vi "Create Humi Tag.vi"(8 "error in (no error)":errorcluster, 11 "CVT Tags to Create":T1) -> (0 "error out":errorcluster, 3 "CVT CFG Out":T1)   [LabVIEW 2016, in "CVT.lvlib"]
uses:
  <vilib>/NI/Current Value Table/Type Defs/File Format.ctl
  <vilib>/NI/Current Value Table/Type Defs/Single Tag.ctl
  <vilib>/NI/Current Value Table/Type Defs/Data Types.ctl
  <vilib>/NI/Current Value Table/Type Defs/Tag Grouping set.ctl
  CVT.lvlib
  <vilib>/NI/Current Value Table/Current Value Table.lvlib
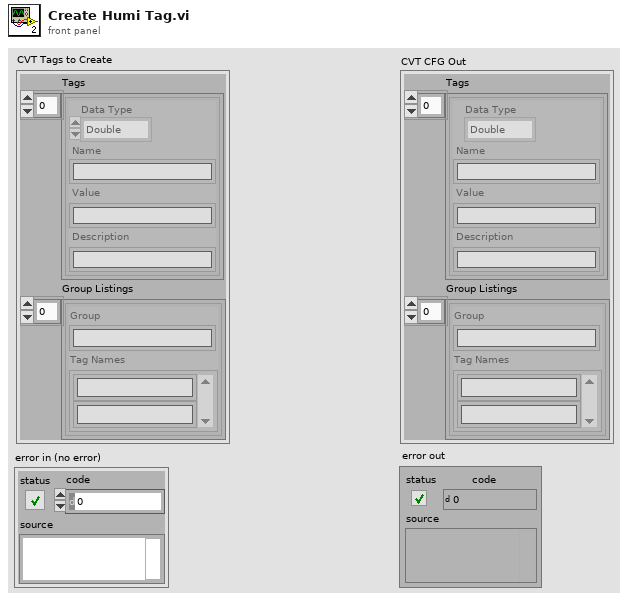
[diagram p1: front panel]
types:
  T1 = typedef "CVT.lvlib/Current Value Table.lvlib/File Format.ctl" = cluster{"Tags":T2[], "Group Listings":T4[]}
  T2 = typedef "CVT.lvlib/Current Value Table.lvlib/Single Tag.ctl" = cluster{"Data Type":T3, "Name":string, "Value":string, "Description":string}
  T3 = typedef "CVT.lvlib/Current Value Table.lvlib/Data Types.ctl" = enum16{"Double", "Single", "I64", "I32", "I16", "I8", "U64", "U32", "U16", "U8", "String", "Boolean", "Array of U8", "Array of U16", "Array of U32", "Array of U64", "Array of I64", "Array of I32", "Array of I16", "Array of I8", "Array of Double", "Array of Single", "Array of Boolean", "Array of String"}
  T4 = typedef "CVT.lvlib/Current Value Table.lvlib/Tag Grouping set.ctl" = cluster{"Group":string, "Tag Names":string[]}
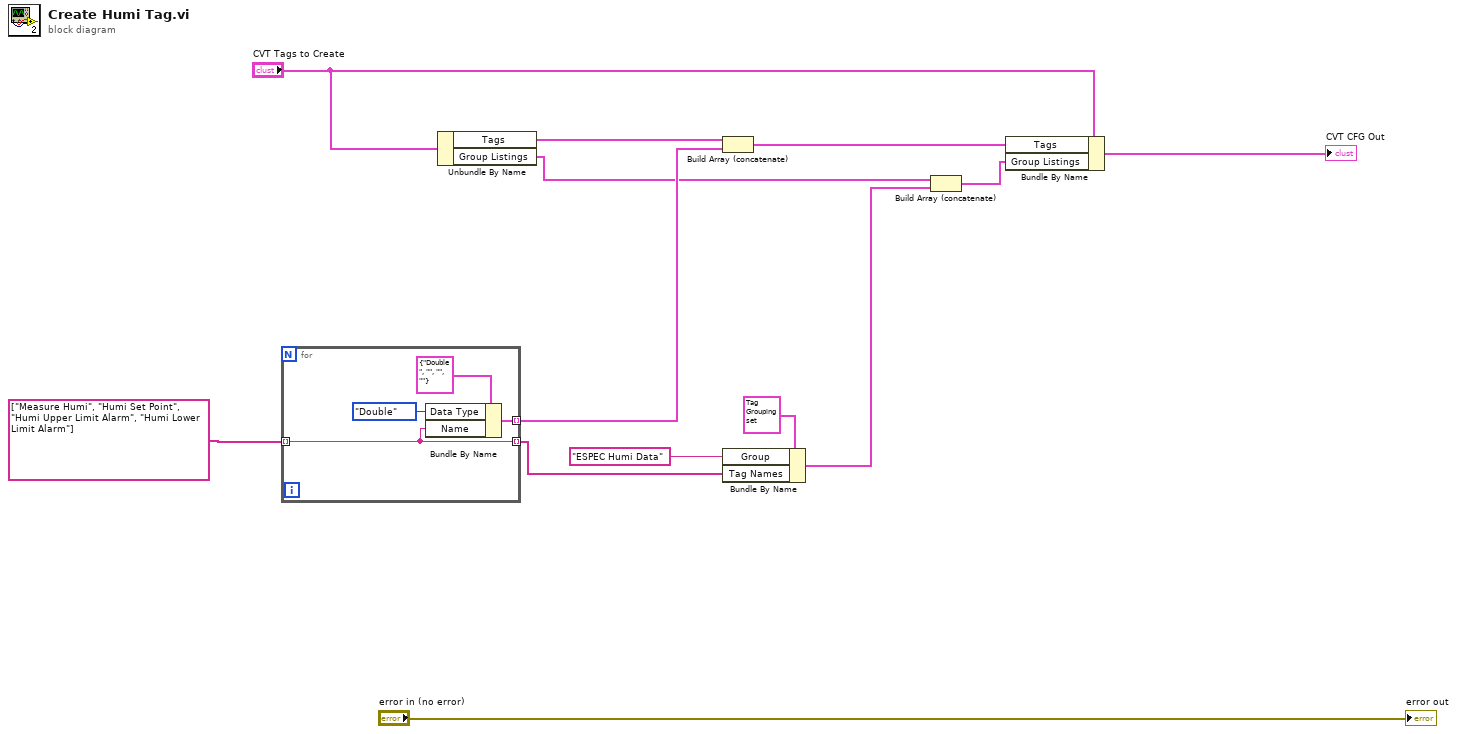
[diagram p0: block diagram]
diagram:
  n1 = for {
    tunnel: string[] ["Measure Humi", "Humi Set Point", "Humi Upper Limit Alarm", "Humi Lower Limit Alarm"] -> [w15] mode=indexing
    tunnel: [w16] -> w6 mode=indexing
    tunnel: [w15] -> w9 mode=indexing
    n2 = Bundle By Name(cluster=T2 {"Data Type"=enum."Double", "Name"="", "Value"="", "Description"=""} ("Tag"), "Data Type"=Data_Types."Double", "Name"=w15) -> (w16:T2)
  }
  n3 = Unbundle By Name("CVT Tags to Create") -> ("Tags"=w7:T2[], "Group Listings"=w4:T4[])
  n4 = Build Array (concatenate)(w7, w6) -> (w5:T2[])
  n5 = Bundle By Name(cluster=T4 {"Group"="Analog Output", "Tag Names"=["AO_0", "AO_1", "AO_2", "AO_3"]} ("Tag Grouping"), "Group"="ESPEC Humi Data", "Tag Names"=w9) -> (w12:T4)
  n6 = Build Array (concatenate)(w4, w12) -> (w3:T4[])
  n7 = Bundle By Name(cluster="CVT Tags to Create", "Tags"=w5, "Group Listings"=w3) -> (→"CVT CFG Out":T1)
  "error out" <- "error in (no error)"
